vi "FPGA IO with LRS.vi"() -> ()   [LabVIEW 2012]
uses:
  <vilib>/rvi/eio/common/nirviEmuClasses.ctl
  <vilib>/rvi/FXPMathLib/FxpDiv/subVIs/nifxpmath_Div_SimConfig.ctl
  <vilib>/rvi/Emulation/niFpgaSctlEmulationGetInTimedLoop.vi
  <vilib>/rvi/Emulation/niFpgaSctlEmulationGlobalWrite.vi
  <vilib>/rvi/eio/common/nirviEmuTemplateMethod_errors.vi
  <vilib>/rvi/FXPMathLib/FxpDiv/simVIs/DllFxpDivTemp_sub.vi
  <vilib>/rvi/eio/common/nirviEmuTemplateMethod_noerrors.vi
  <vilib>/rvi/Memory/Memory_Emulation/nirvimemoryEmulationManagerCache_GetValue.vi
  <vilib>/rvi/Memory/Memory_Emulation/niFpgaMemoryEmulationValidateCache.vi
  <vilib>/rvi/DataTransferAndStorage/Container/Common/niFpgaContainerGetUniqueNameForEmu.vi
  <vilib>/rvi/Memory/Memory_Emulation/nirvimemoryEmulationManagerCache_InsertValue.vi
  <vilib>/rvi/Memory/Memory_Emulation/nirvimemoryEmulationManagerCache_SetValue.vi
  <vilib>/rvi/Emulation/niFpgaSctlEmulationResourceMgr.vi
  <vilib>/rvi/interface/RandomDataEmulation/nirviRandomDataFPGAFIFO.vi
  <vilib>/rvi/interface/RandomDataEmulation/niFpgaRandomDataHandleErrors.vi
  <vilib>/rvi/Memory/Memory_Emulation/niFpgaMemoryEmulationCacheClearOnFirstRun.vi
  <vilib>/rvi/Memory/Memory_Emulation/nirvimemoryEmulationManagerCache_MakeExclusive.vi
  <vilib>/rvi/Memory/Memory_Emulation/nirvimemoryEmulationManagerCache_ReleaseExclusive.vi
  <vilib>/Utility/error.llb/Clear Errors.vi
  <vilib>/eio/EIOGrowableMethodNode/genericMethod/EIOGrowableMethodNode.xnode
  <vilib>/rvi/eio/nirviEIOMethodImplementation/nirviEIOMethodImplementation.xnode
  <vilib>/rvi/eio/nirviErrorMerge/nirviErrorMerge.xnode
  <vilib>/rvi/FXPMathLib/FxpMul/XNode/nifxpmath_Multiplier.xnode
  <vilib>/rvi/FXPMathLib/FxpAdd/XNode/nifxpmath_Add.xnode
  <vilib>/rvi/FXPMathLib/FxpDiv/XNode/nifxpmath_Div.xnode
  <vilib>/rvi/DataTransferAndStorage/Container/XNode/niFpgaContainer.xnode
  <vilib>/rvi/DataTransferAndStorage/Register/Emulation/niFpgaRegisterEmulation.vi
  <vilib>/rvi/interface/RandomDataEmulation/nirviRandomDataFpgaReadWriteTemplate.vi
  <vilib>/rvi/Memory/Memory_Emulation/nirvimemoryEmulation.vi
  <vilib>/eio/EIONode/EIONode.xnode
  <vilib>/rvi/FXPMathLib/sim/FxpSim.dll
panel:
  in  "Stop":bool
  out "loop rate":u32
  out "time between":u32
  out "Timed Out":bool
  out "Stopped":bool
  out "Error Out":errorcluster
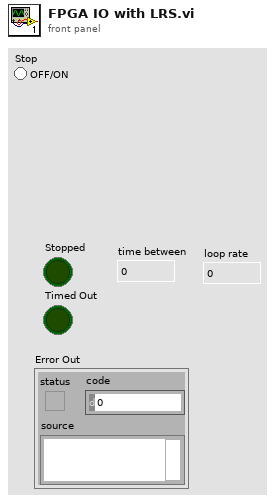
[diagram p1: front panel]
types:
  T1 = typedef "nirviEmuClasses.ctl" = enum16{"IO Read", "IO Write", "Method", "Property Read", "Property Write"}
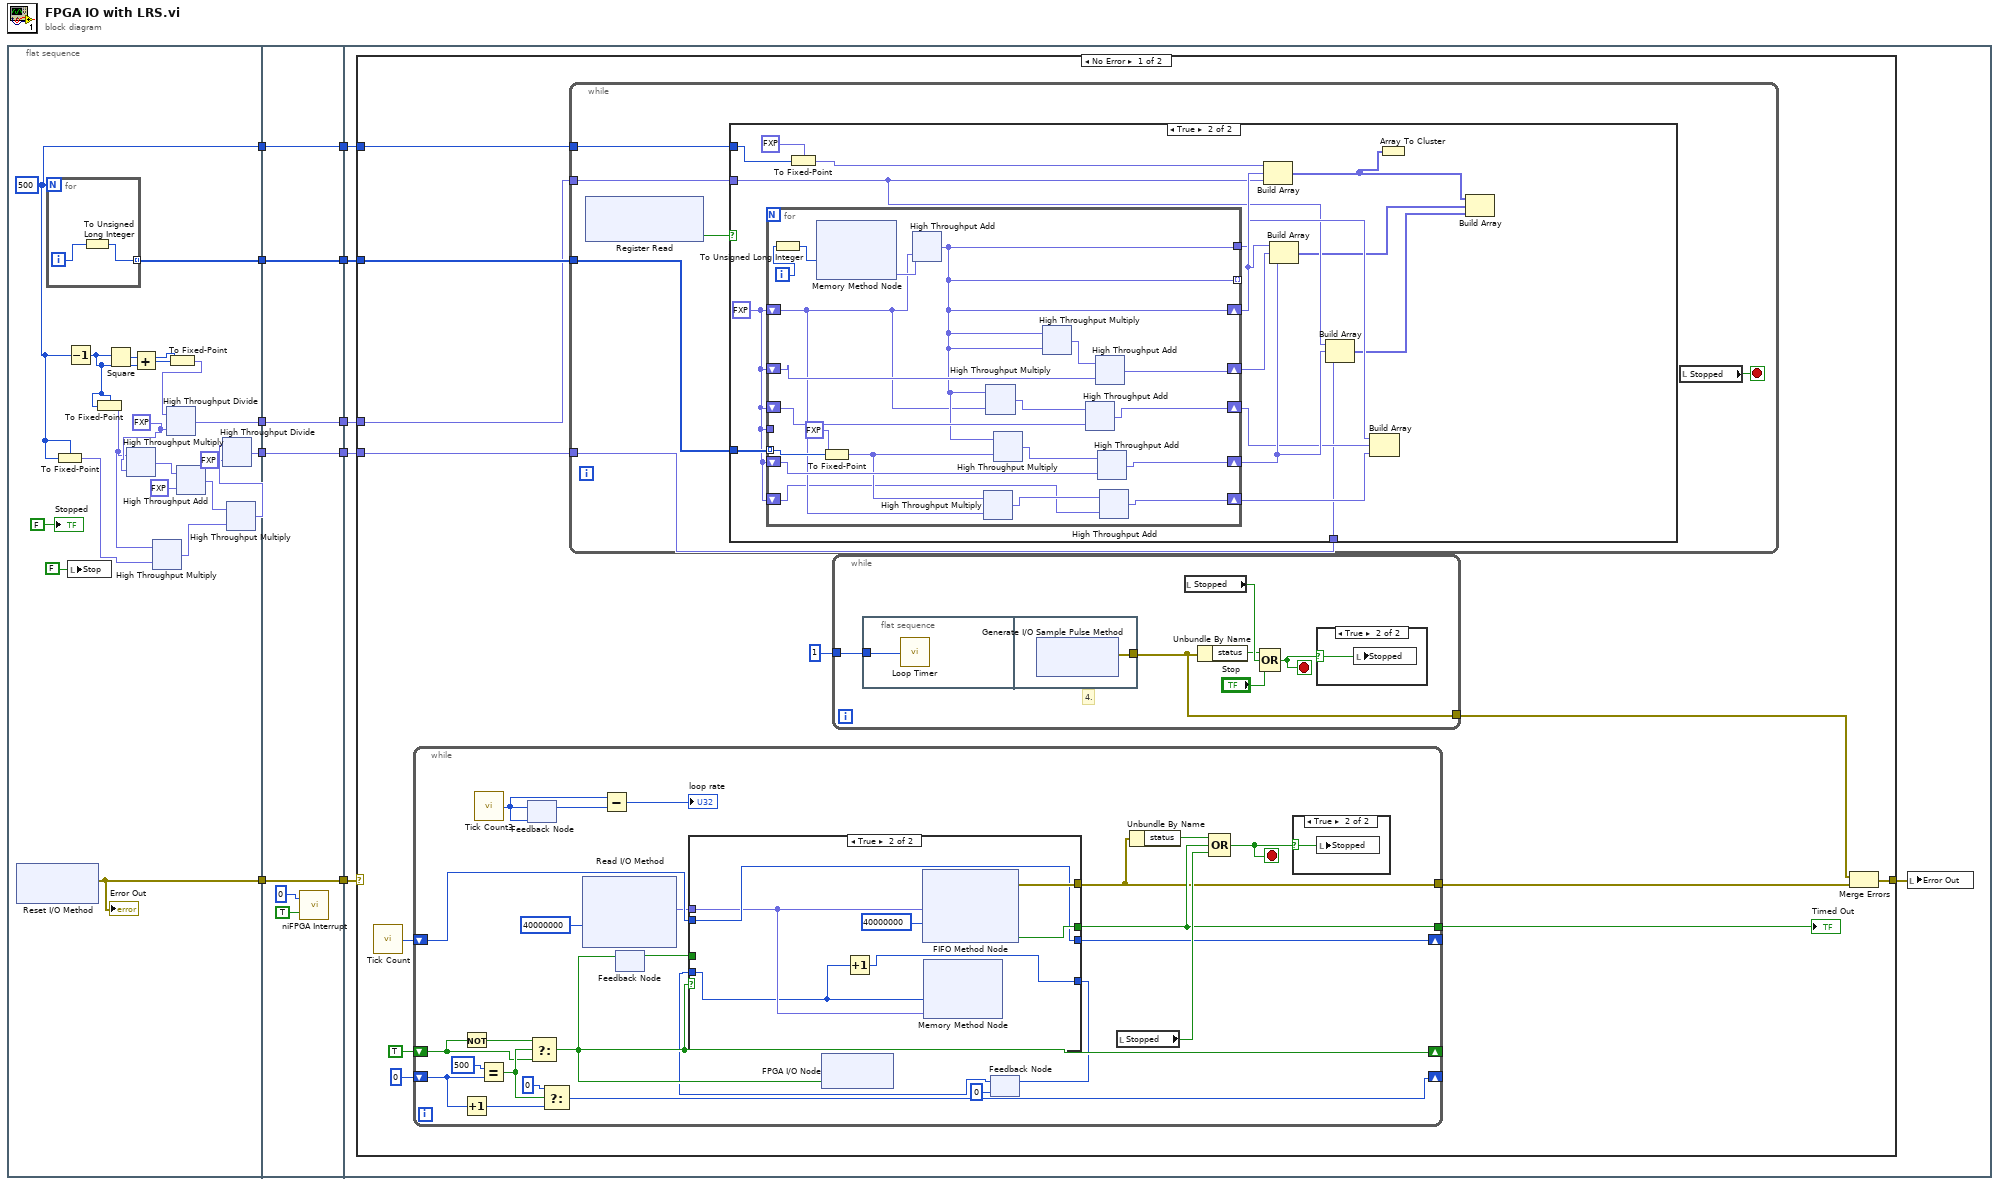
[diagram p0: block diagram]
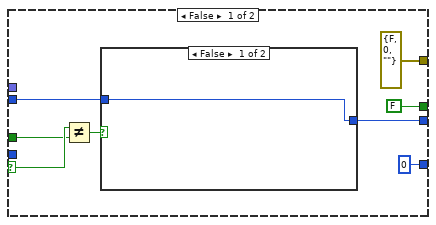
[diagram p4: hidden frame]
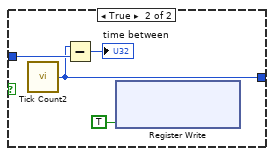
[diagram p5: hidden frame]
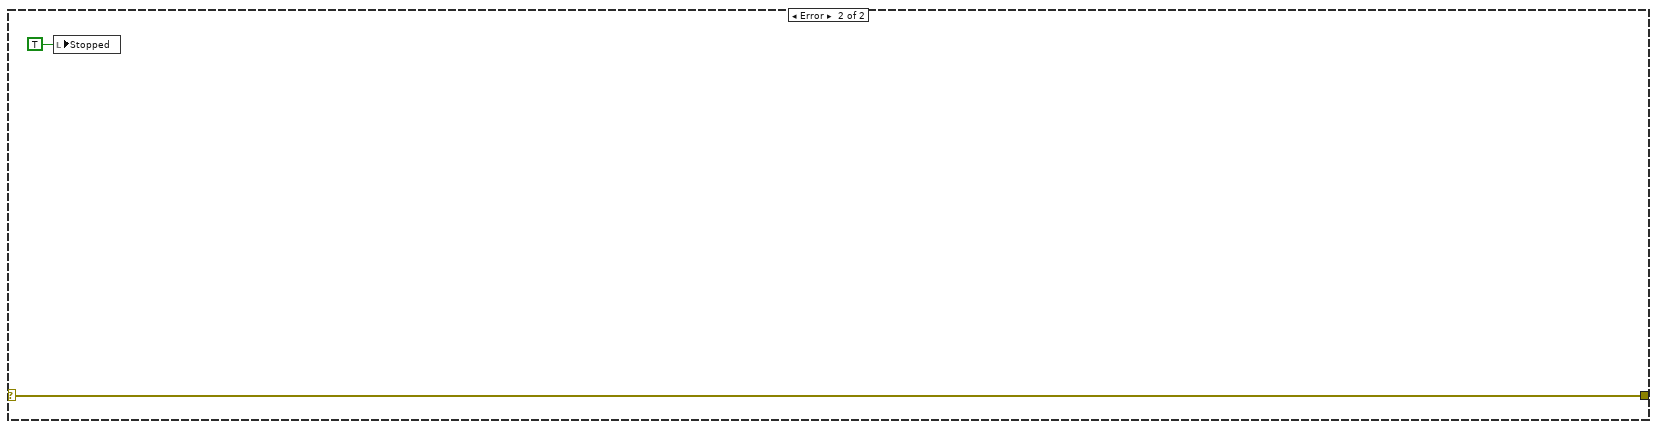
[diagram p7: hidden frame]
diagram:
  n1 = flat-sequence {
    tunnel: [w29] -> w10
    tunnel: [w27] -> w7
    tunnel: [w16] -> w5
    tunnel: [w20] -> w3
    tunnel: [w11] -> w1
    tunnel: w10 -> [w136]
    tunnel: [w136] -> w9
    tunnel: [w135] -> w8
    tunnel: w7 -> [w135]
    tunnel: [w134] -> w6
    tunnel: w5 -> [w134]
    tunnel: [w133] -> w4
    tunnel: w3 -> [w133]
    tunnel: [w132] -> w2
    tunnel: w1 -> [w132]
    tunnel: w9 -> [w144]
    tunnel: w8 -> [w142]
    tunnel: w6 -> [w141]
    tunnel: w4 -> [w140]
    tunnel: w2 -> [w139]
    frame #0 {
      w22 = fxp<+,8,8> 2.0 ("y")
      w16 = 500
      n2 = xnode "Reset I/O Method"() -> ("error out"=w29:errorcluster)  [unwired: 2 in, 1 out]
      "Error Out" <- w29
      n3 = for {
        N: w16 -> [_]
        tunnel: [w85] -> w27 mode=indexing
        i -> [w86]
        n4 = To Unsigned Long Integer(number=w86) -> (unsigned 32bit integer=w85:u32)
      }
      n5 = To Fixed-Point(fixed-point type=w16, number=w16) -> (fixed-point=w15:fxp<+/-,32,32>)
      n6 = Decrement(x=w16) -> (x-1=w23:i32)
      n7 = local write "Stop"(FALSE ("Stop")) -> ()
      n8 = To Fixed-Point(fixed-point type=w23, number=w23) -> (fixed-point=w17:fxp<+/-,32,32>)
      n9 = Square(x=w23) -> (x^2=w25:i32)
      n10 = xnode ("High Throughput Multiply")("x"=w17, "y"=w22) -> ("x*y"=w21:fxp<+/-,64,40>)
      n11 = Add(x=w25, y=w23) -> (x+y=w26:i32)
      n12 = xnode ("High Throughput Multiply")("x"=w17, "y"=w15) -> ("x*y"=w14:fxp<+/-,64,40>)
      n13 = To Fixed-Point(fixed-point type=w26, number=w25) -> (fixed-point=w24:fxp<+/-,32,32>)
      n14 = xnode "High Throughput Divide"("x"=w24, "y"=w22) -> ("x/y"=w20:fxp<+/-,64,40>)
      n15 = xnode ("High Throughput Add")("x"=w21, "y"=fxp<+/-,64,40> 1.0) -> ("x+y"=w18:fxp<+/-,64,40>)
      n16 = xnode ("High Throughput Multiply")("x"=w18, "y"=w14) -> ("x*y"=w13:fxp<+/-,64,40>)
      n17 = xnode "High Throughput Divide"("x"=w13, "y"=fxp<+,8,8> 6.0) -> ("x/y"=w11:fxp<+/-,64,40>)
      "Stopped" <- FALSE ("Stopped")
    }
    frame #1 {
      n18 = call <vilib>:"niFPGA Interrupt.vi"("Wait Until Cleared (F)"=TRUE ("Wait Until Cleared"), "IRQ Number (0)"=u8 0 ("IRQ Number")) -> ()  [unwired: 1 in]
    }
    frame #2 {
      n19 = case shown="No Error" w144 {
        selector: w144 -> [_ w333]
        tunnel: [w156 w333] -> w143
        tunnel: w142 -> [w148 _]
        tunnel: w141 -> [w147 _]
        tunnel: w140 -> [w146 _]
        tunnel: w139 -> [w145 _]
        frame No Error {
          n20 = call "Tick Count"() -> ("Tick Count(uSec)"=w149:u32)
          n21 = while {
            shift-right: [w215] -> _
            shift-left: u32 0 ("Number of Samples") -> [w218]
            tunnel: [w220] -> w152
            shift-right: [w202] -> _
            shift-left: TRUE ("Timed Out") -> [w212]
            tunnel: [w211] -> w150
            shift-right: [w208] -> _
            shift-left: w149 -> [w209]
            stop <- w221 stop-if-true
            n22 = Not(x=w212) -> (.not. x?=w213:bool)
            n23 = Increment(x=w218) -> (x+1=w217:u32)
            n24 = call "Tick Count3"() -> ("Tick Count(uSec)"=w207:u32)
            n25 = Equal?(x=u32 500 ("y"), y=w218) -> (x = y?=w214:bool)
            n26 = feedback-in #1(w207) -> ()
            n27 = feedback #1(w207) -> (w206:u32)
            n28 = Select(t=w213, s=w214, f=w212) -> (s? t:f=w202:bool)
            n29 = Select(t=u32 0 ("Number of Samples"), s=w214, f=w217) -> (s? t:f=w215:u32)
            n30 = xnode "Read I/O Method"("Timeout"=40000000) -> ("CRD Las In"=w203:fxp<+/-,24,5>)  [unwired: 2 in, 3 out]
            n31 = Subtract(x=w207, y=w206) -> (x-y=→"loop rate":u32)
            n32 = feedback-in #2(w202) -> ()
            n33 = feedback #2() -> (w210:bool)  [unwired: 1 in]
            n34 = xnode "FPGA I/O Node"("CRDS"=w202) -> ()  [unwired: 1 in, 1 out]
            n35 = feedback #3(u32 0 ("Address")) -> (w199:u32)
            n36 = case shown="True" w202 {
              selector: w202 -> [w264 _]
              tunnel: [errorcluster {"status"=FALSE, "code"=0, "source"=""} ("error out") w278] -> w211
              tunnel: [FALSE ("Timed Out?") w277] -> w220
              tunnel: w210 -> [w263 _]
              tunnel: w209 -> [w262 w276]
              tunnel: [w261 w276] -> w208
              tunnel: w203 -> [_ w274]
              tunnel: [u32 0 w272] -> w201
              tunnel: w199 -> [_ w273]
              frame False {
                n37 = Not Equal?(x=w264, y=w263) -> (x != y?=w260:bool)
                n38 = case shown="False" w260 {
                  tunnel: w262 -> [w267 w271]
                  tunnel: [w267 w270] -> w261
                  frame False {
                  }
                  frame True {
                    n39 = call "Tick Count2"() -> ("Tick Count(uSec)"=w270:u32)
                    n40 = Subtract(x=w270, y=w271) -> (x-y=→"time between":u32)
                    n41 = xnode ("Register Write")("Data"=TRUE) -> ()  [unwired: 1 in, 1 out]
                  }
                }
              }
              frame True {
                n42 = Increment(x=w273) -> (x+1=w272:u32)
                n43 = xnode ("FIFO Method Node")("Element"=w274, "Timeout"=40000000) -> ("Timed Out?"=w277:bool, "error out"=w278:errorcluster)  [unwired: 2 in, 1 out]
                n44 = xnode ("Memory Method Node")("Address"=w273, "Data"=w274) -> ()  [unwired: 1 in, 1 out]
              }
            }
            n45 = feedback-in #3(w201) -> ()
            n46 = local read "Stopped"() -> (w222:bool)
            n47 = Unbundle By Name(w211) -> ("status"=w223:bool)
            n48 = Compound Arithmetic op=OR(w223, w220, w222) -> (w221:bool)
            n49 = case shown="True" w221 {
              selector: w221 -> [_ w258]
              frame False {
              }
              frame True {
                n50 = local write "Stopped"(w258) -> ()
              }
            }
          }
          "Timed Out" <- w152
          n51 = while {
            tunnel: w148 -> [w160]
            tunnel: w147 -> [w159]
            tunnel: w146 -> [w158]
            tunnel: w145 -> [w157]
            stop <- w162 stop-if-true
            n52 = xnode ("Register Read")() -> ("Data"=w161:bool)  [unwired: 1 in, 1 out]
            n53 = case shown="True" w161 {
              tunnel: w160 -> [_ w178]
              tunnel: w159 -> [_ w176]
              tunnel: w158 -> [_ w167]
              tunnel: w157 -> [_ w166]
              frame False {
              }
              frame True {
                w177 = fxp<+/-,64,40> 0.0 ("x+y")
                n54 = for {
                  shift-right: [w188] -> w173
                  shift-left: w177 -> [w183]
                  tunnel: [w188] -> _ mode=indexing
                  tunnel: [w188] -> w170
                  shift-right: [w196] -> w172
                  shift-left: w177 -> [w195]
                  shift-right: [w192] -> w169
                  shift-left: w177 -> [w194]
                  tunnel: w178 -> [w189] mode=indexing
                  tunnel: w177 -> [_]
                  shift-right: [w185] -> w171
                  shift-left: w177 -> [w186]
                  shift-right: [w180] -> w168
                  shift-left: w177 -> [w181]
                  i -> [w191]
                  n55 = To Unsigned Long Integer(number=w191) -> (unsigned 32bit integer=w190:u32)
                  n56 = xnode ("Memory Method Node")("Address"=w190) -> ("Data"=w198:fxp<+/-,24,5>)  [unwired: 1 in, 1 out]
                  n57 = To Fixed-Point(fixed-point type=fxp<+,32,32> 0.0, number=w189) -> (fixed-point=w184:fxp<+,32,32>)
                  n58 = xnode ("High Throughput Add")("x"=w198, "y"=w183) -> ("x+y"=w188:fxp<+/-,64,40>)
                  n59 = xnode ("High Throughput Multiply")("x"=w184, "y"=w183) -> ("x*y"=w182:fxp<+/-,64,40>)
                  n60 = xnode ("High Throughput Multiply")("x"=w188, "y"=w183) -> ("x*y"=w193:fxp<+/-,64,40>)
                  n61 = xnode ("High Throughput Multiply")("x"=w188, "y"=w184) -> ("x*y"=w187:fxp<+/-,64,40>)
                  n62 = xnode ("High Throughput Multiply")("x"=w188, "y"=w188) -> ("x*y"=w197:fxp<+/-,64,40>)
                  n63 = xnode ("High Throughput Add")("x"=w193, "y"=w194) -> ("x+y"=w192:fxp<+/-,64,40>)
                  n64 = xnode ("High Throughput Add")("x"=w197, "y"=w195) -> ("x+y"=w196:fxp<+/-,64,40>)
                  n65 = xnode ("High Throughput Add")("x"=w187, "y"=w186) -> ("x+y"=w185:fxp<+/-,64,40>)
                  n66 = xnode ("High Throughput Add")("x"=w182, "y"=w181) -> ("x+y"=w180:fxp<+/-,64,40>)
                }
                n67 = To Fixed-Point(fixed-point type=fxp<+/-,64,40> 0.0, number=w176) -> (fixed-point=w174:fxp<+/-,64,40>)
                n68 = Build Array(w174, w173, w167) -> (w163:fxp<+/-,64,40>[])
                n69 = Build Array(w173, w172, w171) -> (w165:fxp<+/-,64,40>[])
                n70 = Build Array(w167, w171, w166) -> (w164:fxp<+/-,64,40>[])
                n71 = Build Array(w170, w169, w168) -> ()  [unwired: 1 out]
                n72 = Array To Cluster(array=w163) -> ()  [unwired: 1 out]
                n73 = Build Array(w163, w165, w164) -> ()  [unwired: 1 out]
              }
            }
            n74 = local read "Stopped"() -> (w162:bool)
          }
          n75 = while {
            tunnel: u32 1 ("Sample Period (uSec)") -> [w284]
            tunnel: [w281] -> w153
            stop <- w280 stop-if-true
            # "4."
            n76 = flat-sequence {
              tunnel: w284 -> [w286]
              tunnel: [w287] -> w281
              frame #0 {
                n77 = call "Loop Timer"("Count(uSec)"=w286) -> ()  [unwired: 1 out]
              }
              frame #1 {
                n78 = xnode "Generate I/O Sample Pulse Method"() -> ("error out"=w287:errorcluster)  [unwired: 2 in, 1 out]
              }
            }
            n79 = local read "Stopped"() -> (w283:bool)
            n80 = Unbundle By Name(w281) -> ("status"=w282:bool)
            n81 = Compound Arithmetic op=OR(w282, w283, "Stop") -> (w280:bool)
            n82 = case shown="True" w280 {
              selector: w280 -> [_ w285]
              frame False {
              }
              frame True {
                n83 = local write "Stopped"(w285) -> ()
              }
            }
          }
          n84 = Merge Errors(w153, w150) -> (w156:errorcluster)
        }
        frame Error {
          n85 = local write "Stopped"(TRUE ("Stopped")) -> ()
        }
      }
      n86 = local write "Error Out"(w143) -> ()
    }
  }
